vi "Manual.vi"() -> ()   [LabVIEW 2016]
uses:
  Ctls/Open2.ctl
  Ctls/Exit.ctl
  Ctls/Snap.ctl
  Ctls/Analysis.ctl
  Ctls/Grab.ctl
  Ctls/Save.ctl
  Ctls/Add.ctl
  Ctls/Remove.ctl
  Ctls/New.ctl
  <vilib>/userdefined/High Color/IMAQdx.ctl
  Ctls/Manual Steps.ctl
  <vilib>/vision/driver/IMAQdx.llb/IMAQdx Acquisition Mode.ctl
  <vilib>/vision/driver/IMAQdx.llb/IMAQdx Buffer Number Mode.ctl
  <vilib>/vision/driver/NI_Vision_Acquisition_Software.lvlib
panel:
  in  "相机选择":T1="acA1600-20gc"
  in  "新建模板":T2
  in  "Remove":T3
  in  "Add":T4
  in  "机种：":string(combo)="PCB"
  out "Centre":dbl[][](array[numeric])
  in  "保存":T5
  out "Rotate":dbl
  in  "下侧卡槽参数：":T6
  in  "上侧卡槽参数：":T7
  in  "摄像":T8
  in  "分析图片":T9
  in  "拍照":T10
  in  "退出":T11
  in  "打开图片":T12
  out "Image":T13(plugin-control)
  # "PCB 抓取工站视觉手动界面"
  # "V1.0"
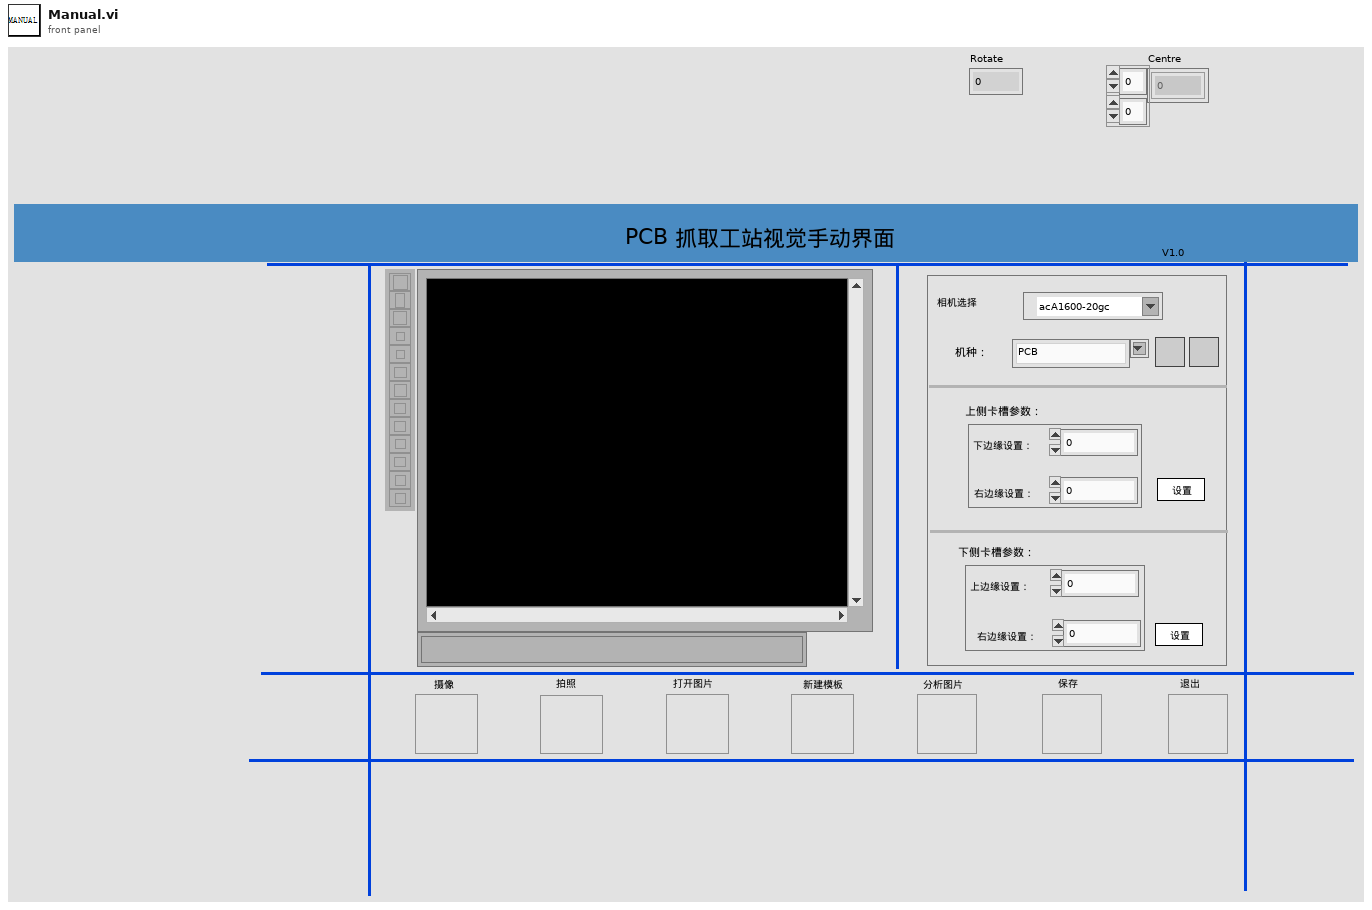
[diagram p1: front panel]
types:
  T1 = typedef "IMAQdx.ctl" = refnum<k21>
  T2 = typedef "New.ctl" = bool
  T3 = typedef "Remove.ctl" = bool
  T4 = typedef "Add.ctl" = bool
  T5 = typedef "Save.ctl" = bool
  T6 = cluster{"Boolean":bool, "Cluster":cluster{"上边缘设置：":i32, "右边缘设置：":i32}}
  T7 = cluster{"Boolean":bool, "Cluster":cluster{"下边缘设置：":i32, "右边缘设置：":i32}}
  T8 = typedef "Grab.ctl" = bool
  T9 = typedef "Analysis.ctl" = bool
  T10 = typedef "Snap.ctl" = bool
  T11 = typedef "Exit.ctl" = bool
  T12 = typedef "Open2.ctl" = bool
  T13 = typedef "IMAQ Image.ctl" = refnum<image>
  T14 = typedef "Manual Steps.ctl" = enum16{"Nothing", "Initial", "Snap", "Grab", "Openpic", "BuildTemp", "TopParameter", "BottomParameter", "Analysis", "Save", "Exit"}
  T15 = typedef "NI_Vision_Acquisition_Software.lvlib/IMAQdx Acquisition Mode.ctl" = enum32{"One Shot", "Continuous"}
  T16 = typedef "NI_Vision_Acquisition_Software.lvlib/IMAQdx Buffer Number Mode.ctl" = enum32{"Next", "Last", "Buffer Number", "Every", "Last New"}
  T17 = cluster{"Boolean":bool, "Cluster":cluster{"上边缘Top设置：":i32, "左侧边Top设置： ":i32}}
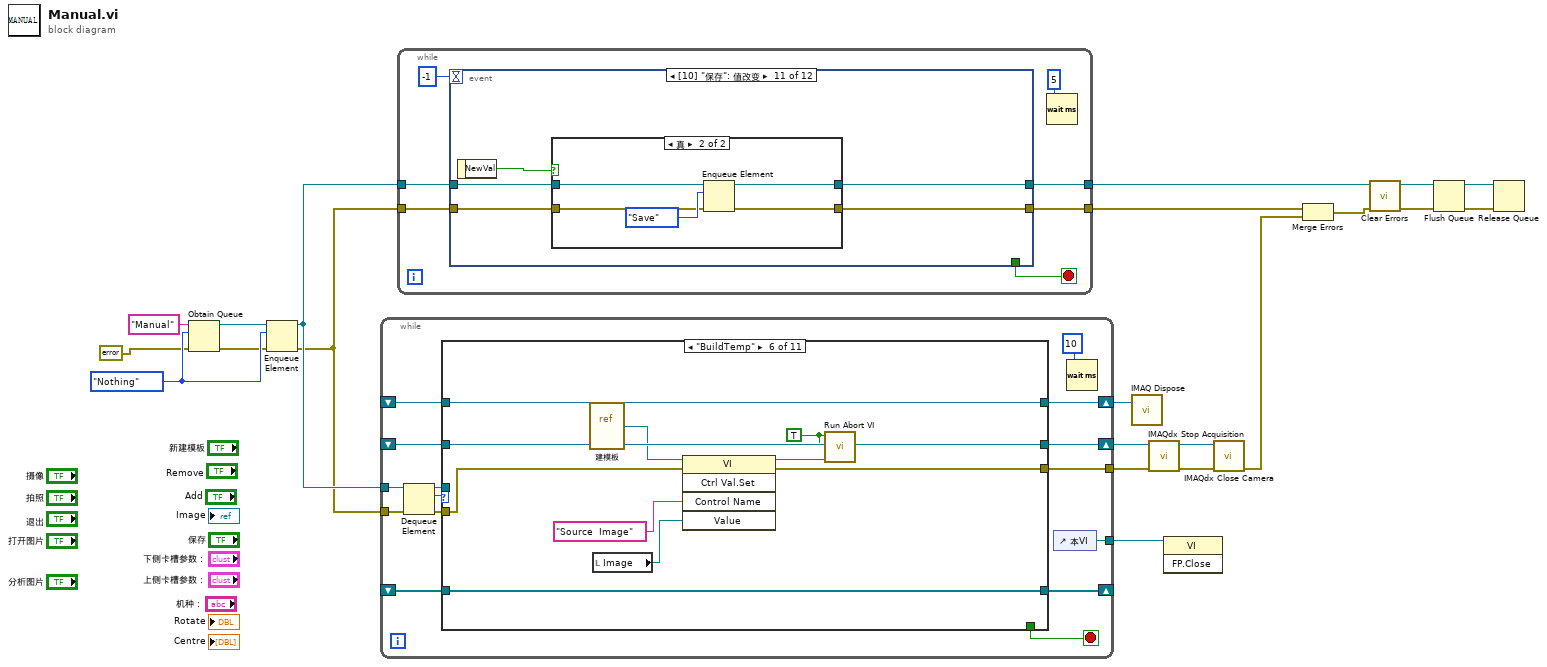
[diagram p0: block diagram]
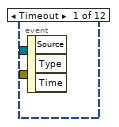
[diagram p2: hidden frame]
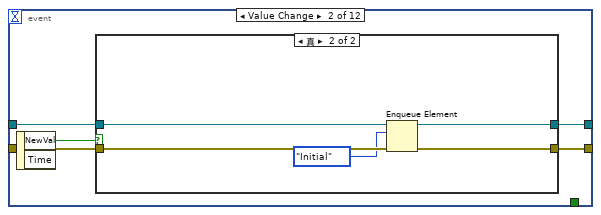
[diagram p3: hidden frame]
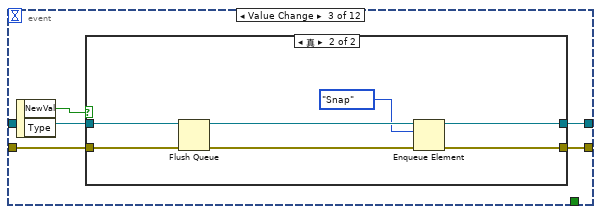
[diagram p5: hidden frame]
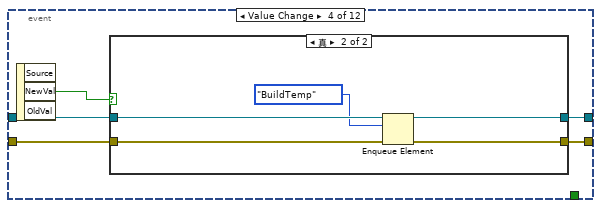
[diagram p7: hidden frame]
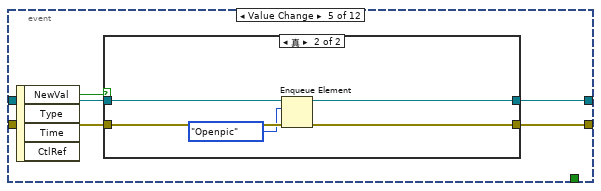
[diagram p9: hidden frame]
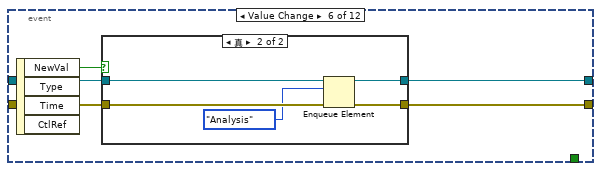
[diagram p11: hidden frame]
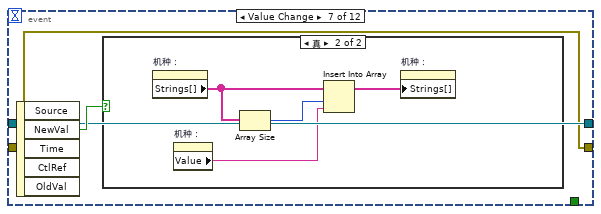
[diagram p13: hidden frame]
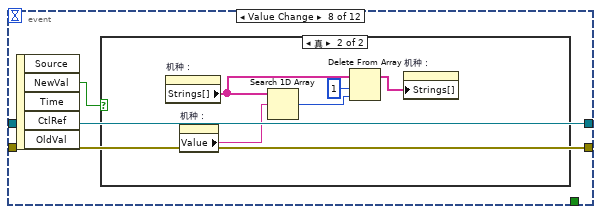
[diagram p15: hidden frame]
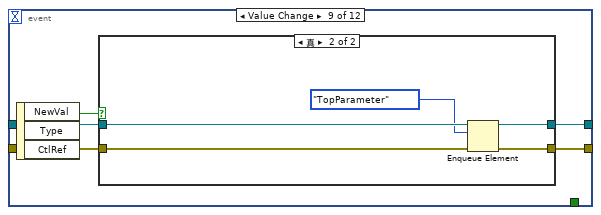
[diagram p17: hidden frame]
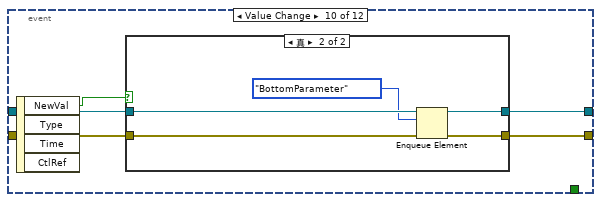
[diagram p19: hidden frame]
diagram:
  w18 = Manual_Steps."Nothing"
  n1 = Obtain Queue(name (unnamed)="Manual", element data type=w18, error in (no error)=errorcluster {"status"=FALSE, "code"=0, "source"=""}) -> (queue out=w19:refnum<queue>, error out=w17:errorcluster)  [unwired: 2 in, 1 out]
  n2 = Enqueue Element(queue=w19, element=w18, error in (no error)=w17) -> (queue out=w15:refnum<queue>, error out=w14:errorcluster)  [unwired: 1 in, 1 out]
  n3 = while {
    tunnel: w15 -> [w35]
    tunnel: w14 -> [w34]
    tunnel: [w31] -> w4
    shift-right: [w29] -> w9
    shift-left: _ -> [w28]
    shift-right: [w24] -> w8
    shift-left: _ -> [w27]
    tunnel: [w23] -> w1
    shift-right: [w21] -> _
    shift-left: _ -> [w22]
    stop <- w30 stop-if-true
    n4 = Dequeue Element(queue=w35, error in (no error)=w34) -> (queue out=w26:refnum<queue>, element=w33:T14, error out=w32:errorcluster)  [unwired: 1 in, 1 out]
    n5 = case shown="\"BuildTemp\"" w33 {
      tunnel: w32 -> [w41 w67 w82 w96 w110 w118 w135 w150 w164 w179 w187]
      tunnel: [w41 w68 w81 w92 w103 w117 w134 w149 w158 w178 w186] -> w31
      tunnel: [_ _ _ _ _ _ _ _ _ _ TRUE] -> w30
      tunnel: [w43 w73 w84 w94 w114 w124 w138 w152 w170 w181 w190] -> w29
      tunnel: w28 -> [w43 _ w85 w97 w114 w124 w138 w152 w170 w181 w190]
      tunnel: w27 -> [w42 _ w86 w98 w113 w123 w137 w151 w169 w180 w189]
      tunnel: w26 -> [_ w66 _ w91 _ _ _ _ _ _ _]
      tunnel: [w42 w70 w83 w95 w113 w123 w137 w151 w169 w180 w189] -> w24
      tunnel: w22 -> [_ w56 w80 w89 w105 w115 w125 w139 w153 w171 w188]
      tunnel: [w36 w56 w80 w89 w105 w115 w125 w139 w153 w171 w188] -> w21
      frame "Nothing" {
        n6 = call "Path.vi"() -> ("ini"=w40:path)  [unwired: 11 in]
        n7 = Strip Path(path=w40) -> (stripped path=w39:path)  [unwired: 1 out]
        n8 = List Folder(path=w39, pattern="*.png" ("模式")) -> (filenames=w37:string[])  [unwired: 2 in, 3 out]
        n9 = for {
          tunnel: w37 -> [w52] mode=indexing
          tunnel: w39 -> [w53]
          tunnel: [w50] -> w36 mode=indexing
          i -> [w46]
          n10 = Number To Decimal String(number=w46) -> (decimal integer string=w45:string)  [unwired: 1 in]
          n11 = Build Path(base path=w53, name or relative path=w52) -> (appended path=w51:path)
          n12 = Concatenate Strings("MaTem" ("Image Name"), w45) -> (w49:string)
          n13 = call "IMAQ Create"("Image Name"=w49) -> ("New Image"=w47:T13)  [unwired: 4 in, 1 out]
          n14 = call "IMAQ Read Image And Vision Info"("File Path"=w51, "Image"=w47) -> ("Image Out"=w50:T13)  [unwired: 7 in, 2 out]
          n15 = Wait (ms)(milliseconds to wait=u32 2 ("等待时间（毫秒）")) -> ()  [unwired: 1 out]
        }
      }
      frame "Initial" {
        w55 = enum16{"CH1", "CH2", "CH3", "CH4"}."CH1" ("通道")
        w54 = u32 57600 ("baud rate")
        w69 = T17 {"Boolean"=FALSE, "Cluster"={"上边缘Top设置："=0, "左侧边Top设置： "=0}} ("右相机找边参数：")
        n16 = Enqueue Element(queue=w66, element=Manual_Steps."Grab", error in (no error)=w67) -> (error out=w62:errorcluster)  [unwired: 1 in, 2 out]
        n17 = call "自制光源控制.vi"("通道"=w55, "VISA In"=refnum<visa-resource-name> "COM1", "错误输入"=w62, "操作模式"=enum16{"打开", "关闭", "设置"}."打开", "baud rate"=w54) -> ("错误输出"=w58:errorcluster)  [unwired: 4 in, 2 out]
        n18 = call "自制光源控制.vi"("通道"=w55, "VISA In"=refnum<visa-resource-name> "COM1", "错误输入"=w58, "亮度"="255", "操作模式"=enum16{"打开", "关闭", "设置"}."设置", "baud rate"=w54) -> ("错误输出"=w57:errorcluster)  [unwired: 3 in, 2 out]
        n19 = property on="上侧卡槽参数：" class="Clust (严格)"("Value"=w69) -> ()  [unwired: 2 in, 2 out]
        n20 = property on="下侧卡槽参数：" class="Clust (严格)"("Value"=w69) -> ()  [unwired: 2 in, 2 out]
        n21 = call <vilib>:"IMAQdx Open Camera.vi"("error in"=w57, "Session In"="相机选择") -> ("error out"=w74:errorcluster, "Session Out"=w75:T1)  [unwired: 8 in]
        n22 = call <vilib>:"IMAQdx Configure Acquisition.vi"("error in"=w74, "Number of Buffers"=u32 1, "Continuous?"=IMAQdx_Acquisition_Mode."Continuous", "Session In"=w75) -> ("error out"=w72:errorcluster, "Session Out"=w71:T1)  [unwired: 6 in]
        n23 = call <vilib>:"IMAQdx Start Acquisition.vi"("error in"=w72, "Session In"=w71) -> ("error out"=w68:errorcluster, "Session Out"=w70:T1)  [unwired: 8 in]
        n24 = call "IMAQ Create"("Image Name"="Came") -> ("New Image"=w73:T13)  [unwired: 4 in, 1 out]
      }
      frame "Snap" {
        n25 = call <vilib>:"IMAQdx Get Image2.vi"("Buffer Number Mode (Next)"=IMAQdx_Buffer_Number_Mode."Buffer Number", "error in"=w82, "Buffer Number In"=u32 0, "Image In"=w85, "Session In"=w86) -> ("error out"=w81:errorcluster, "Image Out"=w84:T13, "Session Out"=w83:T1)  [unwired: 3 in, 1 out]
        n26 = local write "Image"(w84) -> ()
      }
      frame "Grab" {
        n27 = call <vilib>:"IMAQdx Get Image2.vi"("Buffer Number Mode (Next)"=IMAQdx_Buffer_Number_Mode."Buffer Number", "error in"=w96, "Buffer Number In"=u32 0, "Image In"=w97, "Session In"=w98) -> ("error out"=w93:errorcluster, "Image Out"=w94:T13, "Session Out"=w95:T1)  [unwired: 3 in, 1 out]
        n28 = local write "Image"(w94) -> ()
        n29 = Enqueue Element(queue=w91, element=Manual_Steps."Grab", error in (no error)=w93) -> (error out=w92:errorcluster)  [unwired: 1 in, 2 out]
      }
      frame "Openpic" {
        n30 = call "IMAQ Create"("Image Name"="Image", "error in (no error)"=w110) -> ("New Image"=w111:T13, "error out"=w109:errorcluster)  [unwired: 3 in]
        n31 = call "File Dialog"("start path"=path "D:/SIEMENS/图片/sd卡槽") -> ("selected path"=w112:path, "error out"=w104:errorcluster)  [unwired: 11 in, 2 out]
        n32 = call "IMAQ ReadFile"("File Path"=w112, "error in (no error)"=w109, "Image"=w111) -> ("error out"=w101:errorcluster, "Image Out"=w108:T13)  [unwired: 4 in, 3 out]
        n33 = local write "Image"(w108) -> ()
        n34 = call <vilib>:"Clear Errors.vi"("error in (no error)"=w104) -> ("error out"=w102:errorcluster)  [unwired: 5 in, 1 out]
        n35 = Merge Errors(w102, w101) -> (w103:errorcluster)
      }
      frame "BuildTemp" {
        w116 = TRUE ("Run?(Default Abort)")
        n36 = vi-ref "建模板.vi"() -> (w122:refnum<vi>)
        n37 = local read "Image"() -> (w119:T13)
        n38 = invoke class="VI" method="Ctrl Val.Set"(reference=w122, error in=w118, "Control Name"="Source  Image", "Value"=w119) -> (reference out=w121:refnum<vi>, error out=w117:errorcluster)  [unwired: 1 in, 3 out]
        n39 = call "Run Abort VI.vi"("VI引用句柄"=w121, "Front Panel Window:Open"=w116, "Run?(Default Abort)"=w116) -> ()  [unwired: 9 in]
      }
      frame "TopParameter" {
        n40 = local read "Image"() -> (w133:T13)
        n41 = property on="上侧卡槽参数：" class="Clust (严格)"() -> ("Value"=w131:T7)  [unwired: 2 in, 2 out]
        n42 = local read "Rotate"() -> (w128:dbl)
        n43 = local read "Centre"() -> (w136:dbl[][])
        n44 = Unbundle By Name(w131) -> ("Cluster"=w130:cluster{"下边缘设置：":i32, "右边缘设置：":i32})
        n45 = Subtract(x=w128, y=90.0) -> (x-y=w126:dbl)
        n46 = call "Generate ROI.vi"("Rotate"=w126, "Cluster"=w130, "Centre"=w136, "error in (no error)"=w135, "Command"=enum16{"Top", "Bottom"}."Top", "Image"=w133) -> ("error out"=w134:errorcluster, "Image Out"=w132:T13)  [unwired: 4 in]
        n47 = local write "Image"(w132) -> ()
      }
      frame "BottomParameter" {
        n48 = local read "Image"() -> (w145:T13)
        n49 = property on="下侧卡槽参数：" class="Clust (严格)"() -> ("Value"=w147:T6)  [unwired: 2 in, 2 out]
        n50 = local read "Rotate"() -> (w142:dbl)
        n51 = Unbundle By Name(w147) -> ("Cluster"=w146:cluster{"上边缘设置：":i32, "右边缘设置：":i32})
        n52 = local read "Centre"() -> (w148:dbl[][])
        n53 = Subtract(x=w142, y=90.0) -> (x-y=w140:dbl)
        n54 = call "Generate ROI.vi"("Rotate"=w140, "Cluster"=w146, "Centre"=w148, "error in (no error)"=w150, "Command"=enum16{"Top", "Bottom"}."Bottom", "Image"=w145) -> ("error out"=w149:errorcluster, "Image Out"=w144:T13)  [unwired: 4 in]
        n55 = local write "Image"(w144) -> ()
      }
      frame "Analysis" {
        n56 = property on="机种：" class="CmbBox"() -> ("Value"=w165:string)  [unwired: 2 in, 2 out]
        n57 = call "Manual Save.vi"("机种"=w165, "Command"=enum16{"Write", "Read"}."Read", "error in (no error)"=w164) -> ("Top Read"=w155:cluster{"下边缘设置：":i32, "右边缘设置：":i32}, "Bottom read"=w156:cluster{"上边缘设置：":i32, "右边缘设置：":i32}, "error out"=w159:errorcluster)  [unwired: 10 in]
        n58 = Bundle By Name(cluster=T17 {"Boolean"=FALSE, "Cluster"={"上边缘Top设置："=0, "左侧边Top设置： "=0}} ("右相机找边参数："), "Cluster"=w155) -> (w157:T17)
        n59 = Bundle By Name(cluster=T17 {"Boolean"=FALSE, "Cluster"={"上边缘Top设置："=0, "左侧边Top设置： "=0}} ("右相机找边参数："), "Cluster"=w156) -> (w167:T17)
        n60 = property on="下侧卡槽参数：" class="Clust (严格)"("Value"=w167) -> ()  [unwired: 2 in, 2 out]
        n61 = property on="上侧卡槽参数：" class="Clust (严格)"("Value"=w157) -> ()  [unwired: 2 in, 2 out]
        n62 = local read "Image"() -> (w161:T13)
        n63 = call "Pic Analysis.vi"("Image in"=w161, "Bottom"=w156, "Top"=w155, "error in"=w159, "Temp"=w153) -> ("Image"=w162:T13, "Centre"=w154:dbl[][], "Angle"=w160:sgl, "错误输出"=w158:errorcluster)  [unwired: 5 in, 2 out]
        n64 = local write "Rotate"(w160) -> ()
        n65 = local write "Image"(w162) -> ()
        n66 = local write "Centre"(w154) -> ()
      }
      frame "Save" {
        n67 = property on="上侧卡槽参数：" class="Clust (严格)"() -> ("Value"=w177:T7)  [unwired: 2 in, 2 out]
        n68 = property on="机种：" class="CmbBox"() -> ("Value"=w175:string)  [unwired: 2 in, 2 out]
        n69 = property on="下侧卡槽参数：" class="Clust (严格)"() -> ("Value"=w176:T6)  [unwired: 2 in, 2 out]
        n70 = Unbundle By Name(w177) -> ("Cluster"=w174:cluster{"下边缘设置：":i32, "右边缘设置：":i32})
        n71 = Unbundle By Name(w176) -> ("Cluster"=w173:cluster{"上边缘设置：":i32, "右边缘设置：":i32})
        n72 = call "Manual Save.vi"("机种"=w175, "Command"=enum16{"Write", "Read"}."Write", "error in (no error)"=w179, "Top"=w174, "Bottom"=w173) -> ("error out"=w178:errorcluster)  [unwired: 8 in, 2 out]
      }
      frame "Exit" {
        n73 = call "自制光源控制.vi"("通道"=enum16{"CH1", "CH2", "CH3", "CH4"}."CH1", "VISA In"=refnum<visa-resource-name> "COM1", "错误输入"=w187, "操作模式"=enum16{"打开", "关闭", "设置"}."关闭", "baud rate"=u32 57600) -> ("错误输出"=w186:errorcluster)  [unwired: 4 in, 2 out]
      }
    }
    n74 = control-ref of="本VI"() -> (w23:refnum<vi>)
    n75 = Wait (ms)(milliseconds to wait=u32 10) -> ()  [unwired: 1 out]
  }
  n76 = while {
    tunnel: w15 -> [w197]
    tunnel: w14 -> [w196]
    tunnel: [w195] -> w13
    tunnel: [w194] -> w11
    stop <- w193 stop-if-true
    n77 = event shown="[10] \"保存\": 值改变" {
      selector: _ -> [_ _ _ _ _ _ _ _ _ _ _ _]
      dyn-events: _ -> [_ _ _ _ _ _ _ _ _ _ _ _]
      timeout: -1 -> [_ _ _ _ _ _ _ _ _ _ _ _]
      tunnel: w197 -> [_ w203 w215 w228 w238 w252 w262 w270 w280 w290 w303 w316]
      tunnel: w196 -> [_ w202 w214 w227 w237 w250 w261 w269 w279 w289 w302 w315]
      tunnel: [_ w201 w212 w225 w240 w249 w261 w269 w277 w291 w300 w314] -> w195
      tunnel: [_ w200 w213 w226 w241 w251 w262 w270 w278 w292 w301 w317] -> w194
      tunnel: [_ _ _ _ _ _ _ _ _ _ _ TRUE] -> w193
      event Timeout {
        n78 = event-data() -> ()  [unwired: 1 in, 3 out]
      }
      event Value Change {
        n79 = event-data() -> ("NewVal"=w199:T8)  [unwired: 1 in, 1 out]
        n80 = case shown="真" w199 {
          tunnel: w203 -> [w205 w210]
          tunnel: w202 -> [w204 w209]
          tunnel: [w204 w208] -> w201
          tunnel: [w205 w207] -> w200
          frame False {
          }
          frame True {
            n81 = Enqueue Element(queue=w210, element=Manual_Steps."Initial", error in (no error)=w209) -> (queue out=w207:refnum<queue>, error out=w208:errorcluster)  [unwired: 1 in, 1 out]
          }
        }
      }
      event Value Change {
        n82 = event-data() -> ("NewVal"=w211:T10)  [unwired: 1 in, 1 out]
        n83 = case shown="真" w211 {
          tunnel: w215 -> [w217 w219]
          tunnel: w214 -> [w216 w222]
          tunnel: [w217 w224] -> w213
          tunnel: [w216 w223] -> w212
          frame False {
          }
          frame True {
            n84 = Flush Queue(queue=w219, error in (no error)=w222) -> (queue out=w220:refnum<queue>, error out=w221:errorcluster)  [unwired: 1 out]
            n85 = Enqueue Element(queue=w220, element=Manual_Steps."Snap", error in (no error)=w221) -> (queue out=w224:refnum<queue>, error out=w223:errorcluster)  [unwired: 1 in, 1 out]
          }
        }
      }
      event Value Change {
        n86 = event-data() -> ("NewVal"=w229:T2)  [unwired: 1 in, 2 out]
        n87 = case shown="真" w229 {
          tunnel: w228 -> [w231 w236]
          tunnel: w227 -> [w230 w235]
          tunnel: [w231 w234] -> w226
          tunnel: [w230 w233] -> w225
          frame False {
          }
          frame True {
            n88 = Enqueue Element(queue=w236, element=Manual_Steps."BuildTemp", error in (no error)=w235) -> (queue out=w234:refnum<queue>, error out=w233:errorcluster)  [unwired: 1 in, 1 out]
          }
        }
      }
      event Value Change {
        n89 = event-data() -> ("NewVal"=w239:T12)  [unwired: 1 in, 3 out]
        n90 = case shown="真" w239 {
          tunnel: [w243 w248] -> w241
          tunnel: [w242 w247] -> w240
          tunnel: w238 -> [w243 w246]
          tunnel: w237 -> [w242 w245]
          frame False {
          }
          frame True {
            n91 = Enqueue Element(queue=w246, element=Manual_Steps."Openpic", error in (no error)=w245) -> (queue out=w248:refnum<queue>, error out=w247:errorcluster)  [unwired: 1 in, 1 out]
          }
        }
      }
      event Value Change {
        n92 = event-data() -> ("NewVal"=w253:T9)  [unwired: 1 in, 3 out]
        n93 = case shown="真" w253 {
          tunnel: w252 -> [w255 w260]
          tunnel: [w255 w259] -> w251
          tunnel: w250 -> [w254 w258]
          tunnel: [w254 w257] -> w249
          frame False {
          }
          frame True {
            n94 = Enqueue Element(queue=w260, element=Manual_Steps."Analysis", error in (no error)=w258) -> (queue out=w259:refnum<queue>, error out=w257:errorcluster)  [unwired: 1 in, 1 out]
          }
        }
      }
      event Value Change {
        n95 = event-data() -> ("NewVal"=w263:T4)  [unwired: 1 in, 4 out]
        n96 = case shown="真" w263 {
          frame False {
          }
          frame True {
            n97 = property on="机种：" class="CmbBox"() -> ("Strings[]"=w266:string[])  [unwired: 2 in, 2 out]
            n98 = property on="机种：" class="CmbBox"() -> ("Value"=w265:string)  [unwired: 2 in, 2 out]
            n99 = Array Size(array=w266) -> (size(s)=w267:i32)
            n100 = Insert Into Array(array=w266, index=w267, new element=w265) -> (w264:string[])
            n101 = property on="机种：" class="CmbBox"("Strings[]"=w264) -> ()  [unwired: 2 in, 2 out]
          }
        }
      }
      event Value Change {
        n102 = event-data() -> ("NewVal"=w268:T3)  [unwired: 1 in, 4 out]
        n103 = case shown="真" w268 {
          frame False {
          }
          frame True {
            n104 = property on="机种：" class="CmbBox"() -> ("Strings[]"=w274:string[])  [unwired: 2 in, 2 out]
            n105 = property on="机种：" class="CmbBox"() -> ("Value"=w275:string)  [unwired: 2 in, 2 out]
            n106 = Search 1D Array(1D array=w274, element=w275) -> (index of element=w273:i32)  [unwired: 1 in]
            n107 = Delete From Array(array=w274, length=1 ("长度"), index=w273) -> (array with subset deleted=w271:string[])  [unwired: 1 out]
            n108 = property on="机种：" class="CmbBox"("Strings[]"=w271) -> ()  [unwired: 2 in, 2 out]
          }
        }
      }
      event "上侧卡槽参数：.Boolean": Value Change {
        n109 = event-data() -> ("NewVal"=w276:bool)  [unwired: 1 in, 2 out]
        n110 = case shown="真" w276 {
          tunnel: w280 -> [w282 w287]
          tunnel: w279 -> [w281 w286]
          tunnel: [w282 w285] -> w278
          tunnel: [w281 w284] -> w277
          frame False {
          }
          frame True {
            n111 = Enqueue Element(queue=w287, element=Manual_Steps."TopParameter", error in (no error)=w286) -> (queue out=w285:refnum<queue>, error out=w284:errorcluster)  [unwired: 1 in, 1 out]
          }
        }
      }
      event "下侧卡槽参数：.Boolean": Value Change {
        n112 = event-data() -> ("NewVal"=w288:bool)  [unwired: 1 in, 3 out]
        n113 = case shown="真" w288 {
          tunnel: [w294 w299] -> w292
          tunnel: [w293 w298] -> w291
          tunnel: w290 -> [w294 w297]
          tunnel: w289 -> [w293 w296]
          frame False {
          }
          frame True {
            n114 = Enqueue Element(queue=w297, element=Manual_Steps."BottomParameter", error in (no error)=w296) -> (queue out=w299:refnum<queue>, error out=w298:errorcluster)  [unwired: 1 in, 1 out]
          }
        }
      }
      event Value Change {
        n115 = event-data() -> ("NewVal"=w304:T5)  [unwired: 1 in]
        n116 = case shown="真" w304 {
          tunnel: w303 -> [w306 w310]
          tunnel: w302 -> [w305 w309]
          tunnel: [w306 w308] -> w301
          tunnel: [w305 w307] -> w300
          frame False {
          }
          frame True {
            n117 = Enqueue Element(queue=w310, element=Manual_Steps."Save", error in (no error)=w309) -> (queue out=w308:refnum<queue>, error out=w307:errorcluster)  [unwired: 1 in, 1 out]
          }
        }
      }
      event Value Change {
        n118 = event-data() -> ()  [unwired: 1 in, 4 out]
        n119 = Enqueue Element(queue=w316, element=Manual_Steps."Exit", error in (no error)=w315) -> (queue out=w317:refnum<queue>, error out=w314:errorcluster)  [unwired: 1 in, 1 out]
      }
    }
    n120 = Wait (ms)(milliseconds to wait=u32 5) -> ()  [unwired: 1 out]
  }
  n121 = call "IMAQ Dispose"("Image"=w9) -> ()  [unwired: 5 in, 1 out]
  n122 = call <vilib>:"IMAQdx Stop Acquisition.vi"("error in"=w4, "Session In"=w8) -> ("error out"=w6:errorcluster, "Session Out"=w7:T1)  [unwired: 8 in]
  n123 = invoke class="VI" method="FP.Close"(reference=w1) -> ()  [unwired: 2 in, 3 out]
  n124 = call <vilib>:"IMAQdx Close Camera.vi"("error in"=w6, "Session In"=w7) -> ("error out"=w5:errorcluster)  [unwired: 9 in]
  n125 = Merge Errors(w13, w5) -> (w3:errorcluster)
  n126 = call <vilib>:"Clear Errors.vi"("error in (no error)"=w3) -> ("error out"=w2:errorcluster)  [unwired: 5 in, 1 out]
  n127 = Flush Queue(queue=w11, error in (no error)=w2) -> (queue out=w10:refnum<queue>, error out=w12:errorcluster)  [unwired: 1 out]
  n128 = Release Queue(queue=w10, error in (no error)=w12) -> ()  [unwired: 1 in, 3 out]
